vi "Destroy.vi"(0 "reference in":refnum<class "TimedDoor2.lvclass">, 5 "error in (no error)":errorcluster) -> (14 "reference out":refnum<class "TimedDoor2.lvclass">, 19 "error out":errorcluster)   [LabVIEW 2020, in "TimedDoor2.lvclass"]
uses:
  TimedDoor2.lvclass
  Door_class/Door.lvclass
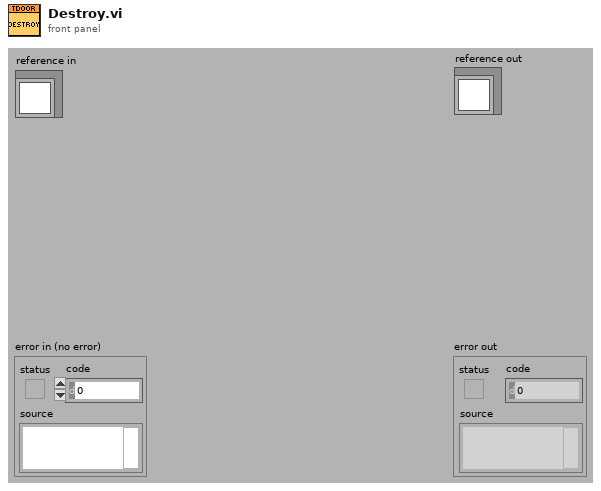
[diagram p1: front panel]
types:
  T1 = typedef "TimedDoor2.lvclass/ObjectAttributes.ctl" = cluster{"Attribute1":dbl}
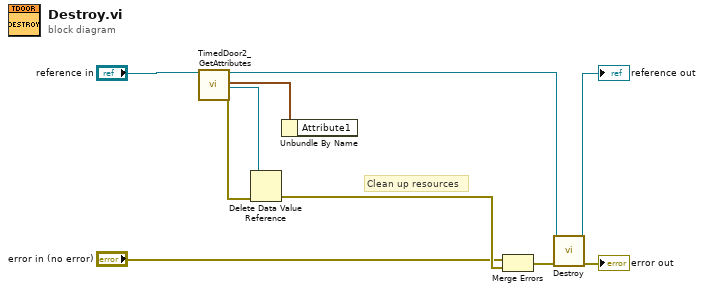
[diagram p0: block diagram]
diagram:
  # "Clean up resources"
  n1 = call "TimedDoor2_GetAttributes.vi"("reference in"="reference in") -> ("reference out"=w2:refnum<class "TimedDoor2.lvclass">, "Data"=w7:T1, "DataRef"=w8:refnum<data-value>, "error out"=w9:errorcluster)  [unwired: 15 in]
  n2 = Delete Data Value Reference(data value reference=w8, error in=w9) -> (error out=w6:errorcluster)  [unwired: 1 out]
  n3 = Unbundle By Name(w7) -> ()  [unwired: 1 out]
  n4 = Merge Errors("error in (no error)", w6) -> (w4:errorcluster)
  n5 = call-parent "Destroy.vi"("reference in"=w2, "error in (no error)"=w4) -> ("reference out"=→"reference out":refnum<class "TimedDoor2.lvclass">, "error out"=→"error out":errorcluster)  [unwired: 16 in]
